vi "Test_for_6581.vi"() -> ()   [LabVIEW 2018]
uses:
  <vilib>/Platform/TimedLoop/XDataNode/timing_clust.ctl
  <vilib>/Platform/TimedLoop/XDataNode/nitl_modes.ctl
  <vilib>/Platform/TimedLoop/XDataNode/wakeup.ctl
  <vilib>/rvi/Emulation/niFpgaSctlEmulationGetInTimedLoop.vi
  <vilib>/rvi/Emulation/niFpgaEmulationReportErrorSimple.vi
  <vilib>/rvi/Emulation/niFpgaGetClockAttributes.vi
  <vilib>/rvi/Emulation/niFpgaCriticalErrorInLSC.vi
  <vilib>/rvi/eio/common/nirviEmuTemplateMethod_errors.vi
  <vilib>/platform/TimedLoop/XDataNode/XDataNode.xnode
  <vilib>/eio/EIONode/EIONode.xnode
  <vilib>/Platform/TimedLoop/XDataNode/XDNodeRunTimeDep.lvlib
panel:
  in  "IO Module\\DDCB_PFI3_Write":bool
  in  "IO Module\\DDCB_PFI2_Write":bool
  in  "IO Module\\DDCB_PFI1_Write":bool
  in  "IO Module\\DDCB_DIO23_Write":bool
  in  "IO Module\\DDCB_DIO22_Write":bool
  in  "IO Module\\DDCB_DIO21_Write":bool
  in  "IO Module\\DDCB_DIO20_Write":bool
  in  "IO Module\\DDCB_DIO19_Write":bool
  in  "IO Module\\DDCB_DIO18_Write":bool
  in  "IO Module\\DDCB_DIO17_Write":bool
  in  "IO Module\\DDCB_DIO16_Write":bool
  in  "IO Module\\DDCB_DIO15_Write":bool
  in  "IO Module\\DDCB_DIO14_Write":bool
  in  "IO Module\\DDCB_DIO13_Write":bool
  in  "IO Module\\DDCB_DIO12_Write":bool
  in  "IO Module\\DDCB_DIO11_Write":bool
  in  "IO Module\\DDCB_DIO10_Write":bool
  in  "IO Module\\DDCB_DIO9_Write":bool
  in  "IO Module\\DDCB_DIO8_Write":bool
  in  "IO Module\\DDCB_DIO7_Write":bool
  in  "IO Module\\DDCB_DIO6_Write":bool
  in  "IO Module\\DDCB_DIO5_Write":bool
  in  "IO Module\\DDCB_DIO4_Write":bool
  in  "IO Module\\DDCB_DIO3_Write":bool
  in  "IO Module\\DDCB_DIO2_Write":bool
  in  "IO Module\\DDCB_DIO1_Write":bool
  in  "IO Module\\DDCB_DIO0_Write":bool
  in  "IO Module\\DDCA_PFI3_Write":bool
  in  "IO Module\\DDCA_PFI2_Write":bool
  in  "IO Module\\DDCA_PFI1_Write":bool
  in  "IO Module\\DDCA_DIO23_Write":bool
  in  "IO Module\\DDCA_DIO22_Write":bool
  in  "IO Module\\DDCA_DIO21_Write":bool
  in  "IO Module\\DDCA_DIO20_Write":bool
  in  "IO Module\\DDCA_DIO19_Write":bool
  in  "IO Module\\DDCA_DIO18_Write":bool
  in  "IO Module\\DDCA_DIO17_Write":bool
  in  "IO Module\\DDCA_DIO16_Write":bool
  in  "IO Module\\DDCA_DIO15_Write":bool
  in  "IO Module\\DDCA_DIO14_Write":bool
  in  "IO Module\\DDCA_DIO13_Write":bool
  in  "IO Module\\DDCA_DIO12_Write":bool
  in  "IO Module\\DDCA_DIO11_Write":bool
  in  "IO Module\\DDCA_DIO10_Write":bool
  in  "IO Module\\DDCA_DIO9_Write":bool
  in  "IO Module\\DDCA_DIO8_Write":bool
  in  "IO Module\\DDCA_DIO7_Write":bool
  in  "IO Module\\DDCA_DIO6_Write":bool
  in  "IO Module\\DDCA_DIO5_Write":bool
  in  "IO Module\\DDCA_DIO4_Write":bool
  in  "IO Module\\DDCA_DIO3_Write":bool
  in  "IO Module\\DDCA_DIO2_Write":bool
  in  "IO Module\\DDCA_DIO1_Write":bool
  in  "IO Module\\DDCA_DIO0_Write":bool
  in  "Стоп":bool
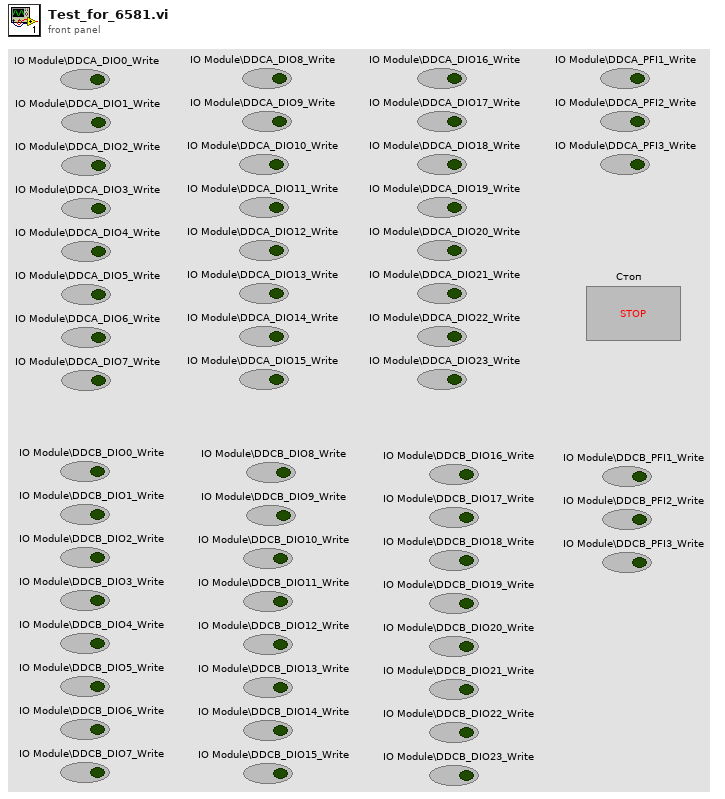
[diagram p1: front panel]
types:
  T1 = typedef "XDNodeRunTimeDep.lvlib/timing_clust.ctl" = cluster{"Expected End [f-1]":u64, "Actual End [f-1]":u64, "Finished Late? [f-1]":bool, "Expected End [i-1]":u64, "Actual End [i-1]":u64, "Finished Late? [i-1]":bool, "Expected Start [i]":u64, "Actual Start [i]":u64, "Expected Start [f]":u64, "Actual Start [f]":u64, "Source Name":string, "Structure Name":string, "Period":i64, "Deadline":i64, "Offset":i64, "Start":i64, "Priority":i32, "Timeout":i32, "Mode":T2, "Wakeup Reason":T3, "Error":errorcluster, "Source Type":string, "Secondary Source Type":string, "Global End Time":u64, "Global Start Time":u64, "Frame Duration":u64, "Iteration Duration":u64, "Assigned CPU":i32, "I/O Scan Engine Mode":u32}
  T2 = typedef "XDNodeRunTimeDep.lvlib/nitl_modes.ctl" = enum32{"No Change", "Process missed periods, maintain original phase", "Discard missed periods, maintain original phase", "Process missed periods, ignore original phase", "Discard missed periods, ignore original phase"}
  T3 = typedef "XDNodeRunTimeDep.lvlib/wakeup.ctl" = enum32{"Normal", "Aborted", "Asynchronous wakeup", "Timing source error", "Timed loop error", "Timeout"}
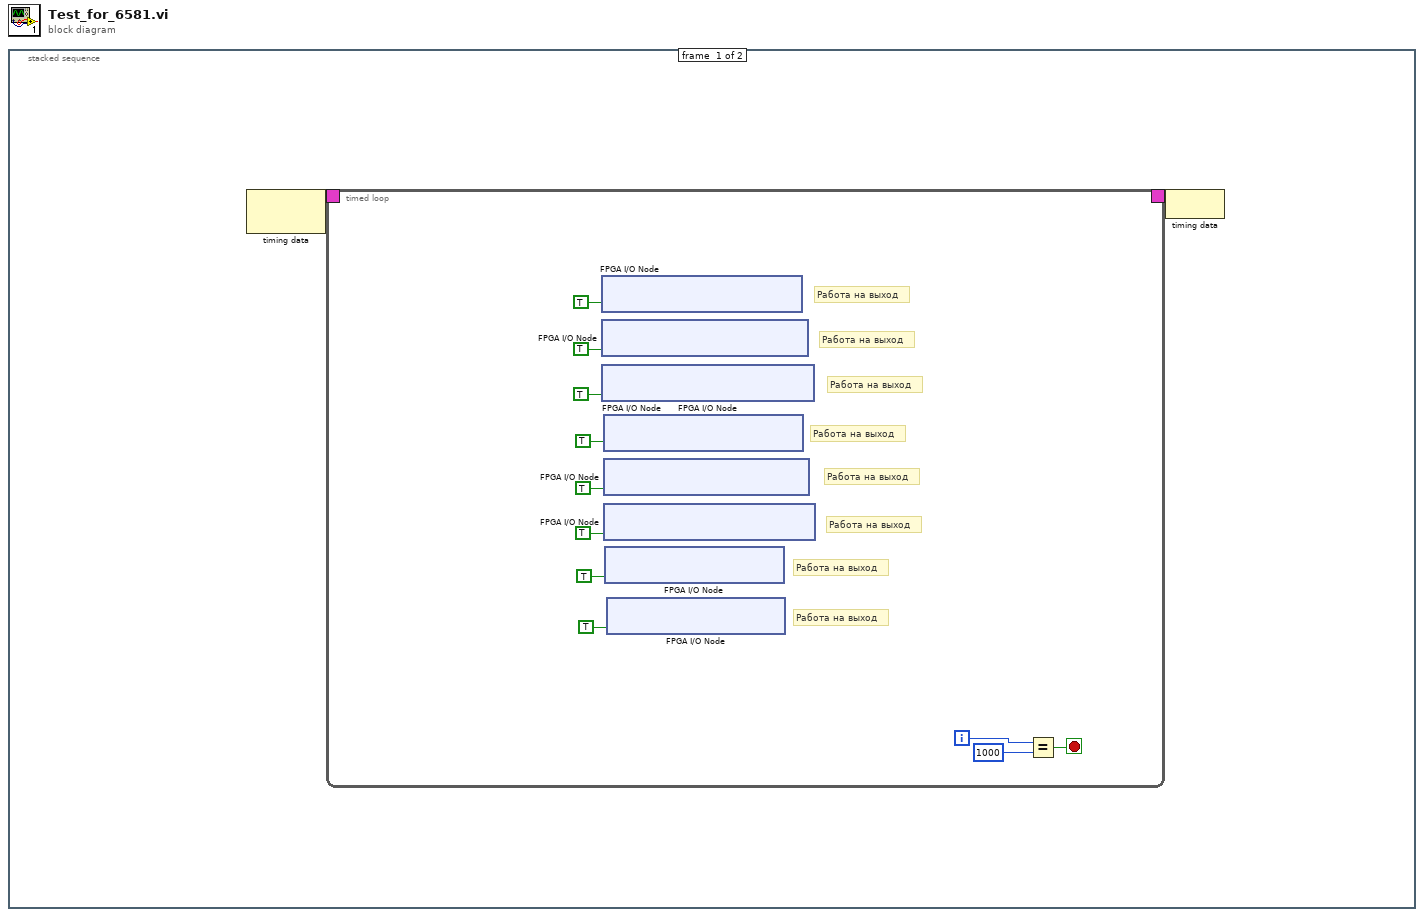
[diagram p0: block diagram]
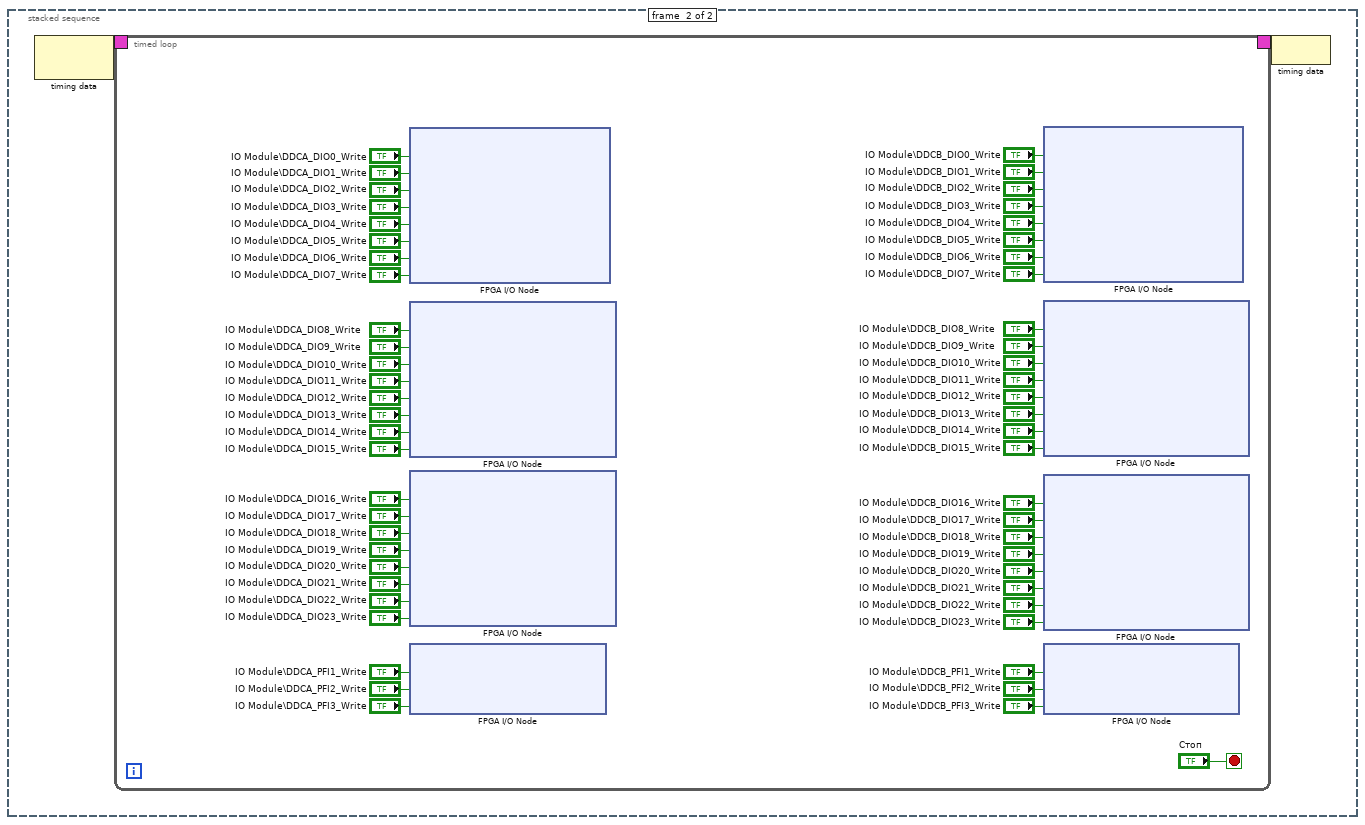
[diagram p2: hidden frame]
diagram:
  n1 = stacked-sequence {
    frame #0 {
      n2 = node-c288() -> (w2:T1)  [unwired: 1 in]
      n3 = timed-loop {
        timing: w2 -> [_]
        timing-out: [_] -> w1
        i -> [w3]
        stop <- w4 stop-if-true
        # "Работа на выход"
        # "Работа на выход"
        # "Работа на выход"
        # "Работа на выход"
        # "Работа на выход"
        # "Работа на выход"
        # "Работа на выход"
        # "Работа на выход"
        n4 = xnode "FPGA I/O Node"("IO Module\\DDCA_DIO0-7_WE"=TRUE ("IO Module\\DDCA_DIO0-7_WE")) -> ()  [unwired: 1 in, 1 out]
        n5 = xnode "FPGA I/O Node"("IO Module\\DDCA_DIO8-15_WE"=TRUE ("IO Module\\DDCA_DIO8-15_WE")) -> ()  [unwired: 1 in, 1 out]
        n6 = xnode "FPGA I/O Node"("IO Module\\DDCA_DIO16-23_WE"=TRUE ("IO Module\\DDCA_DIO8-15_WE")) -> ()  [unwired: 1 in, 1 out]
        n7 = xnode "FPGA I/O Node"("IO Module\\DDCB_DIO0-7_WE"=TRUE ("IO Module\\DDCA_DIO0-7_WE")) -> ()  [unwired: 1 in, 1 out]
        n8 = xnode "FPGA I/O Node"("IO Module\\DDCB_DIO8-15_WE"=TRUE ("IO Module\\DDCA_DIO8-15_WE")) -> ()  [unwired: 1 in, 1 out]
        n9 = xnode "FPGA I/O Node"("IO Module\\DDCB_DIO16-23_WE"=TRUE ("IO Module\\DDCA_DIO8-15_WE")) -> ()  [unwired: 1 in, 1 out]
        n10 = xnode "FPGA I/O Node"("IO Module\\DDCA_PFI_WE"=TRUE ("IO Module\\DDCA_DIO8-15_WE")) -> ()  [unwired: 1 in, 1 out]
        n11 = xnode "FPGA I/O Node"("IO Module\\DDCB_PFI_WE"=TRUE ("IO Module\\DDCA_DIO8-15_WE")) -> ()  [unwired: 1 in, 1 out]
        n12 = Equal?(x=w3, y=1000) -> (x = y?=w4:bool)
      }
      n13 = node-c288(w1) -> ()
    }
    frame #1 {
      n14 = node-c288() -> (w19:T1)  [unwired: 1 in]
      n15 = timed-loop {
        timing: w19 -> [_]
        timing-out: [_] -> w18
        stop <- "Стоп" stop-if-true
        n16 = xnode "FPGA I/O Node"("IO Module\\DDCA_DIO0_Write"="IO Module\\DDCA_DIO0_Write", "IO Module\\DDCA_DIO1_Write"="IO Module\\DDCA_DIO1_Write", "IO Module\\DDCA_DIO2_Write"="IO Module\\DDCA_DIO2_Write", "IO Module\\DDCA_DIO3_Write"="IO Module\\DDCA_DIO3_Write", "IO Module\\DDCA_DIO4_Write"="IO Module\\DDCA_DIO4_Write", "IO Module\\DDCA_DIO5_Write"="IO Module\\DDCA_DIO5_Write", "IO Module\\DDCA_DIO6_Write"="IO Module\\DDCA_DIO6_Write", "IO Module\\DDCA_DIO7_Write"="IO Module\\DDCA_DIO7_Write") -> ()  [unwired: 8 in, 8 out]
        n17 = xnode "FPGA I/O Node"("IO Module\\DDCA_DIO8_Write"="IO Module\\DDCA_DIO8_Write", "IO Module\\DDCA_DIO9_Write"="IO Module\\DDCA_DIO9_Write", "IO Module\\DDCA_DIO10_Write"="IO Module\\DDCA_DIO10_Write", "IO Module\\DDCA_DIO11_Write"="IO Module\\DDCA_DIO11_Write", "IO Module\\DDCA_DIO12_Write"="IO Module\\DDCA_DIO12_Write", "IO Module\\DDCA_DIO13_Write"="IO Module\\DDCA_DIO13_Write", "IO Module\\DDCA_DIO14_Write"="IO Module\\DDCA_DIO14_Write", "IO Module\\DDCA_DIO15_Write"="IO Module\\DDCA_DIO15_Write") -> ()  [unwired: 8 in, 8 out]
        n18 = xnode "FPGA I/O Node"("IO Module\\DDCA_DIO16_Write"="IO Module\\DDCA_DIO16_Write", "IO Module\\DDCA_DIO17_Write"="IO Module\\DDCA_DIO17_Write", "IO Module\\DDCA_DIO18_Write"="IO Module\\DDCA_DIO18_Write", "IO Module\\DDCA_DIO19_Write"="IO Module\\DDCA_DIO19_Write", "IO Module\\DDCA_DIO20_Write"="IO Module\\DDCA_DIO20_Write", "IO Module\\DDCA_DIO21_Write"="IO Module\\DDCA_DIO21_Write", "IO Module\\DDCA_DIO22_Write"="IO Module\\DDCA_DIO22_Write", "IO Module\\DDCA_DIO23_Write"="IO Module\\DDCA_DIO23_Write") -> ()  [unwired: 8 in, 8 out]
        n19 = xnode "FPGA I/O Node"("IO Module\\DDCA_PFI1_Write"="IO Module\\DDCA_PFI1_Write", "IO Module\\DDCA_PFI2_Write"="IO Module\\DDCA_PFI2_Write", "IO Module\\DDCA_PFI3_Write"="IO Module\\DDCA_PFI3_Write") -> ()  [unwired: 3 in, 3 out]
        n20 = xnode "FPGA I/O Node"("IO Module\\DDCB_DIO0_Write"="IO Module\\DDCB_DIO0_Write", "IO Module\\DDCB_DIO1_Write"="IO Module\\DDCB_DIO1_Write", "IO Module\\DDCB_DIO2_Write"="IO Module\\DDCB_DIO2_Write", "IO Module\\DDCB_DIO3_Write"="IO Module\\DDCB_DIO3_Write", "IO Module\\DDCB_DIO4_Write"="IO Module\\DDCB_DIO4_Write", "IO Module\\DDCB_DIO5_Write"="IO Module\\DDCB_DIO5_Write", "IO Module\\DDCB_DIO6_Write"="IO Module\\DDCB_DIO6_Write", "IO Module\\DDCB_DIO7_Write"="IO Module\\DDCB_DIO7_Write") -> ()  [unwired: 8 in, 8 out]
        n21 = xnode "FPGA I/O Node"("IO Module\\DDCB_DIO8_Write"="IO Module\\DDCB_DIO8_Write", "IO Module\\DDCB_DIO9_Write"="IO Module\\DDCB_DIO9_Write", "IO Module\\DDCB_DIO10_Write"="IO Module\\DDCB_DIO10_Write", "IO Module\\DDCB_DIO11_Write"="IO Module\\DDCB_DIO11_Write", "IO Module\\DDCB_DIO12_Write"="IO Module\\DDCB_DIO12_Write", "IO Module\\DDCB_DIO13_Write"="IO Module\\DDCB_DIO13_Write", "IO Module\\DDCB_DIO14_Write"="IO Module\\DDCB_DIO14_Write", "IO Module\\DDCB_DIO15_Write"="IO Module\\DDCB_DIO15_Write") -> ()  [unwired: 8 in, 8 out]
        n22 = xnode "FPGA I/O Node"("IO Module\\DDCB_DIO16_Write"="IO Module\\DDCB_DIO16_Write", "IO Module\\DDCB_DIO17_Write"="IO Module\\DDCB_DIO17_Write", "IO Module\\DDCB_DIO18_Write"="IO Module\\DDCB_DIO18_Write", "IO Module\\DDCB_DIO19_Write"="IO Module\\DDCB_DIO19_Write", "IO Module\\DDCB_DIO20_Write"="IO Module\\DDCB_DIO20_Write", "IO Module\\DDCB_DIO21_Write"="IO Module\\DDCB_DIO21_Write", "IO Module\\DDCB_DIO22_Write"="IO Module\\DDCB_DIO22_Write", "IO Module\\DDCB_DIO23_Write"="IO Module\\DDCB_DIO23_Write") -> ()  [unwired: 8 in, 8 out]
        n23 = xnode "FPGA I/O Node"("IO Module\\DDCB_PFI1_Write"="IO Module\\DDCB_PFI1_Write", "IO Module\\DDCB_PFI2_Write"="IO Module\\DDCB_PFI2_Write", "IO Module\\DDCB_PFI3_Write"="IO Module\\DDCB_PFI3_Write") -> ()  [unwired: 3 in, 3 out]
      }
      n24 = node-c288(w18) -> ()
    }
  }
